vi "Read.vi"(8 "error in (no error)":errorcluster, 9 "Timeout":i32=2000, 10 "NumOfBytes":i32=100, 11 "ClientBase in":refnum<class "TCP.lvclass">) -> (0 "error out":errorcluster, 1 "Length":i32, 2 "Data":string, 3 "ClientBase out":refnum<class "TCP.lvclass">, 4 "Abort":bool)   [LabVIEW 2020, in "TCP.lvlib" / "TCP.lvclass"]
uses:
  TCP.lvclass
  TCP.lvclass/TCP.ctl
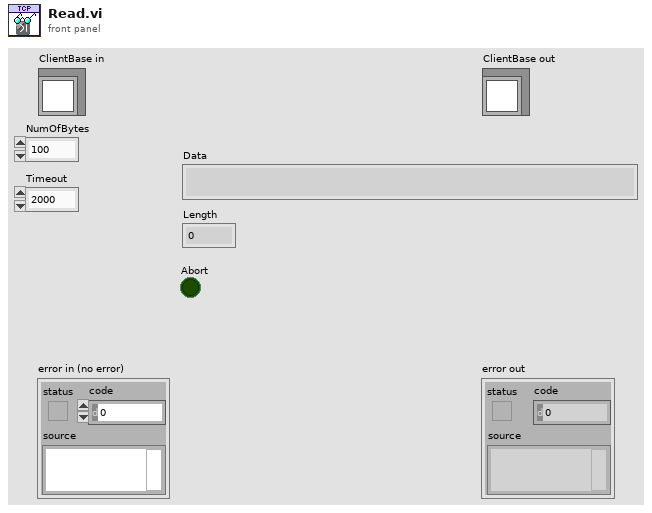
[diagram p1: front panel]
types:
  T1 = enum16{"Standard", "Buffered", "CRLF", "Immediate"}
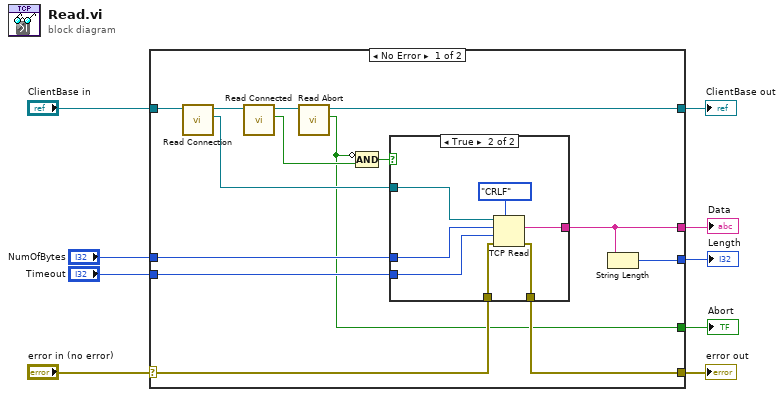
[diagram p0: block diagram]
diagram:
  n1 = case shown="No Error" "error in (no error)" {
    selector: "error in (no error)" -> [w23 w33]
    tunnel: [w22 w33] -> w8
    tunnel: [w12 w32] -> w6
    tunnel: "ClientBase in" -> [w11 w32]
    tunnel: [w21 _] -> w5
    tunnel: [w20 _] -> w4
    tunnel: "Timeout" -> [w18 _]
    tunnel: "NumOfBytes" -> [w17 _]
    tunnel: [w10 _] -> w1
    frame No Error {
      n2 = call "Read Connection.vi"("ClientBase in"=w11) -> ("Connection ID"=w14:refnum<k5>, "ClientBase out"=w16:refnum<class "TCP.lvclass">)  [unwired: 8 in, 1 out]
      n3 = call "Read Connected.vi"("ClientBase in"=w16) -> ("Connected"=w15:bool, "ClientBase out"=w13:refnum<class "TCP.lvclass">)  [unwired: 8 in, 1 out]
      n4 = call "Read Abort.vi"("ClientBase in"=w13) -> ("Abort"=w10:bool, "ClientBase out"=w12:refnum<class "TCP.lvclass">)  [unwired: 8 in, 1 out]
      n5 = Compound Arithmetic op=AND(invert w10, w15) -> (w19:bool)
      n6 = case shown="True" w19 {
        tunnel: w14 -> [_ w31]
        tunnel: w23 -> [w24 w30]
        tunnel: [w24 w29] -> w22
        tunnel: [_ w27] -> w21
        tunnel: w18 -> [_ w26]
        tunnel: w17 -> [_ w25]
        frame False {
        }
        frame True {
          n7 = TCP Read(connection ID=w31, bytes to read=w25, error in (no error)=w30, 7:T1."CRLF" ("mode (standard)"), 9:w26) -> (data out=w27:string, error out=w29:errorcluster)  [unwired: 1 out]
        }
      }
      n8 = String Length(string=w21) -> (length=w20:i32)
    }
    frame Error {
    }
  }
  "error out" <- w8
  "ClientBase out" <- w6
  "Data" <- w5
  "Length" <- w4
  "Abort" <- w1
